vi "test philosopher.vi"() -> ()   [LabVIEW 2023, in "Philosopher.lvlib"]
uses:
  Philosopher.lvlib
  Philosopher/Philosopher.lvclass
  C:/Program Files (x86)/National Instruments/LabVIEW 2023/vi.lib/ActorFramework/Actor/Actor.lvclass
  <vilib>/Utility/miscctls.llb/LVRectTypeDef.ctl
  Philosopher Messages/Take Your Seat Msg/Take Your Seat.lvclass/Take Your Seat.ctl
  <vilib>/ActorFramework/Message Enqueuer/Message Enqueuer.lvclass/Message Enqueuer.ctl
  <vilib>/ActorFramework/Message Enqueuer/Enqueue.vi
  Philosopher Messages/Take Your Seat Msg/Take Your Seat.lvclass
  C:/Program Files (x86)/National Instruments/LabVIEW 2023/vi.lib/ActorFramework/Message/Message.lvclass
  Philosopher Messages/Go to eating Msg/Eat.lvclass
  <vilib>/ActorFramework/Stop Msg/Stop Msg.lvclass
  <vilib>/ActorFramework/Message Priority Queue/Priority Enqueue.vi
  <vilib>/ActorFramework/Actor/Actor.lvclass
panel:
  in  "stop":bool
  in  "Eat":bool
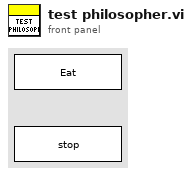
[diagram p1: front panel]
types:
  T1 = typedef "LVRectTypeDef.ctl" = cluster{"Left":i16, "Top":i16, "Right":i16, "Bottom":i16}
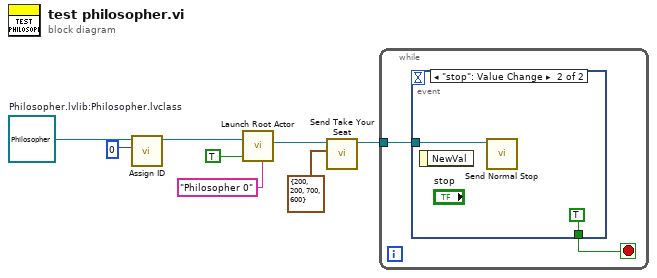
[diagram p0: block diagram]
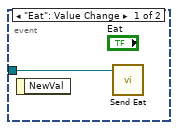
[diagram p2: hidden frame]
diagram:
  w6 = refnum<class "Philosopher.lvclass"> refnum  # Philosopher.lvlib:Philosopher.lvclass
  n1 = call-dynamic "Assign ID.vi"("ID"=0, "Philosopher in"=w6) -> ("Philosopher out"=w5:refnum<class "Philosopher.lvclass">)  [unwired: 8 in, 1 out]
  n2 = call <vilib>:"Launch Root Actor.vi"("Debug Alias"="Philosopher 0", "Open Actor Core front panel? (F)"=TRUE, "Actor"=w5) -> ("Actor's Enqueuer"=w3:refnum<class "Message Enqueuer.lvclass">)  [unwired: 7 in, 1 out]
  n3 = call "Send Take Your Seat.vi"("Front Panel Window:Panel Bounds"=T1 {"Left"=200, "Top"=200, "Right"=700, "Bottom"=600}, "Message Enqueuer"=w3) -> ("Message Enqueuer out"=w2:refnum<class "Message Enqueuer.lvclass">)  [unwired: 8 in, 1 out]
  n4 = while {
    tunnel: w2 -> [w10]
    stop <- w9 stop-if-true
    n5 = event shown="[1] \"stop\": Value Change" {
      selector: _ -> [_ _]
      dyn-events: _ -> [_ _]
      timeout: _ -> [_ _]
      tunnel: w10 -> [w11 w13]
      tunnel: [_ TRUE] -> w9
      event "Eat": Value Change {
        n6 = event-data() -> ()  [unwired: 1 in, 1 out]
        n7 = call "Send Eat.vi"("Message Enqueuer"=w11) -> ()  [unwired: 9 in, 2 out]
      }
      event "stop": Value Change {
        n8 = event-data() -> ()  [unwired: 1 in, 1 out]
        n9 = call <vilib>:"Send Normal Stop.vi"("Message Enqueuer"=w13) -> ()  [unwired: 10 in, 1 out]
      }
    }
  }
